vi "Pulse statistics.vi"() -> ()   [LabVIEW 2015]
uses:
  Library/Shot data.ctl
panel:
  out "Total shots":i32
  out "Numeric Control":i32
  out "Sorted by magnet":cluster{"Array":T1[]}[](array[cluster])
  in  "Lines to skip":i32=2
  out "All Pulses":T1[](array[typedef])
  in  "File Path Control":path=path "G:/Short Pulse Shot history/ShotHistory2012.txt"
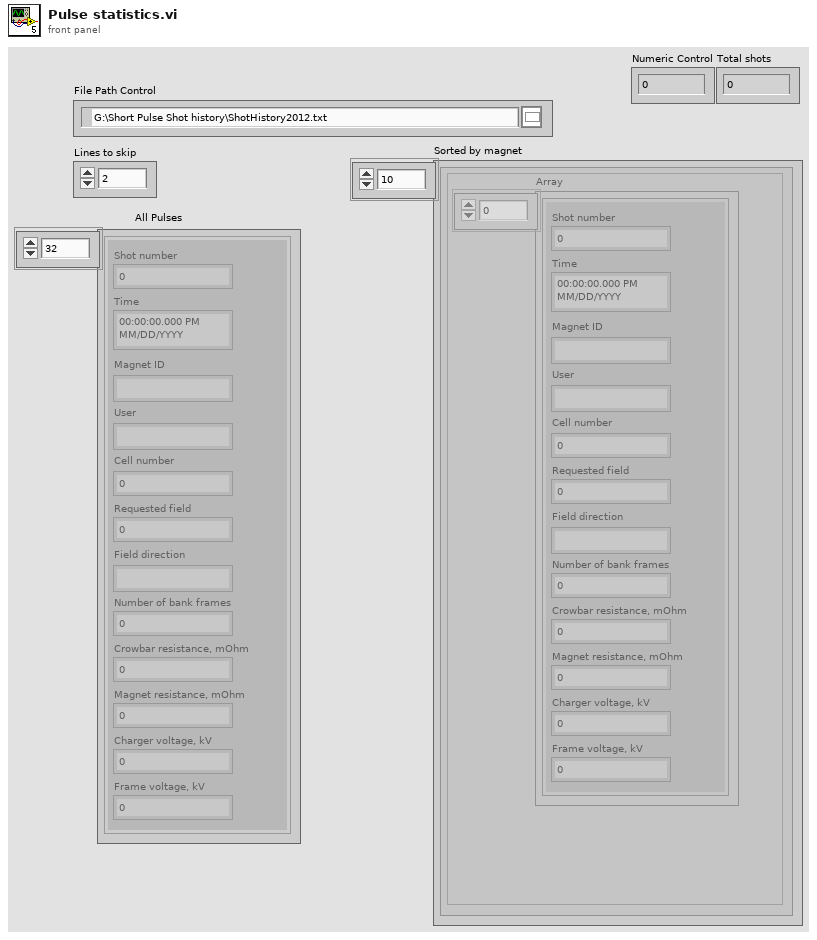
[diagram p1: front panel]
types:
  T1 = typedef "Shot data.ctl" = cluster{"Shot number":i32, "Time":timestamp, "Magnet ID":string, "User":string, "Cell number":i32, "Requested field":dbl, "Field direction":string, "Number of bank frames":i32, "Crowbar resistance, mOhm":dbl, "Magnet resistance, mOhm":dbl, "Charger voltage, kV":dbl, "Frame voltage, kV":dbl}
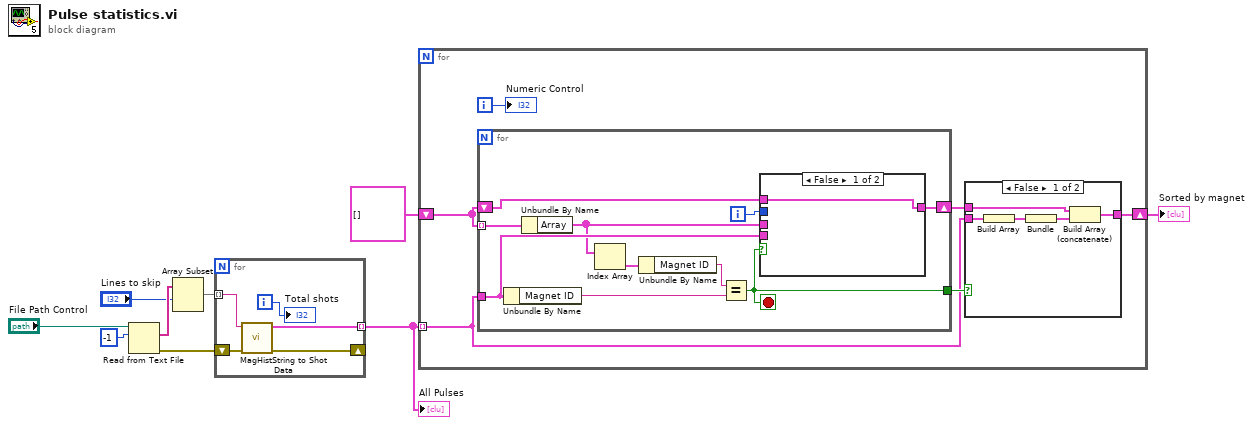
[diagram p0: block diagram]
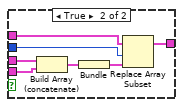
[diagram p3: hidden frame]
diagram:
  n1 = Read from Text File(file (use dialog)="File Path Control", count=-1) -> (text=w7:string[], error out=w6:errorcluster)  [unwired: 2 in, 2 out]
  n2 = Array Subset(array=w7, index="Lines to skip") -> (w5:string[])  [unwired: 1 in]
  n3 = for {
    tunnel: w5 -> [w14] mode=indexing
    shift-right: [w12] -> _
    shift-left: w6 -> [w13]
    tunnel: [w11] -> w3 mode=indexing
    i -> [w10]
    n4 = call "MagHistString to Shot Data.vi"("error in (no error)"=w13, "String"=w14) -> ("error out"=w12:errorcluster, "Shot data"=w11:T1)  [unwired: 8 in]
    "Total shots" <- w10
  }
  "All Pulses" <- w3
  n5 = for {
    tunnel: w3 -> [w16] mode=indexing
    shift-right: [w17] -> w1
    shift-left: cluster{"Array":T1[]}[] [] ("Array") -> [w20]
    i -> [w15]
    n6 = for {
      tunnel: w16 -> [w35]
      tunnel: w20 -> [w27] mode=indexing
      shift-right: [w29] -> w18
      shift-left: w20 -> [w31]
      tunnel: [w28] -> w19
      i -> [w30]
      stop <- w28 stop-if-true
      n7 = Unbundle By Name(w35) -> ("Magnet ID"=w33:string)
      n8 = Unbundle By Name(w27) -> ("Array"=w32:T1[])
      n9 = Index Array(array=w32) -> (element=w36:T1)  [unwired: 1 in]
      n10 = Unbundle By Name(w36) -> ("Magnet ID"=w34:string)
      n11 = Equal?(x=w34, y=w33) -> (x = y?=w28:bool)
      n12 = case shown="False" w28 {
        tunnel: w35 -> [_ w44]
        tunnel: w32 -> [_ w43]
        tunnel: w31 -> [w37 w42]
        tunnel: w30 -> [_ w41]
        tunnel: [w37 w38] -> w29
        frame False {
        }
        frame True {
          n13 = Build Array (concatenate)(w43, w44) -> (w40:T1[])
          n14 = Bundle(w40) -> (w39:cluster{T1[]})  [unwired: 1 in]
          n15 = Replace Array Subset(array=w42, new element=w39, index=w41) -> (w38:cluster{"Array":T1[]}[])
        }
      }
    }
    n16 = case shown="False" w19 {
      tunnel: w18 -> [w23 w26]
      tunnel: [w22 w26] -> w17
      tunnel: w16 -> [w25 _]
      frame False {
        n17 = Build Array(w25) -> (w24:T1[])
        n18 = Bundle(w24) -> (w21:cluster{T1[]})  [unwired: 1 in]
        n19 = Build Array (concatenate)(w23, w21) -> (w22:cluster{"Array":T1[]}[])
      }
      frame True {
      }
    }
    "Numeric Control" <- w15
  }
  "Sorted by magnet" <- w1
